vi "LOX Saturation Lookup.vi"(9 "error in":errorcluster, 11 "Temperature":dbl=-280.0) -> (1 "error out":errorcluster, 2 "Saturation Density":dbl, 3 "Saturation Pressure":dbl)   [LabVIEW 2024]
uses:
  <vilib>/Utility/file.llb/Read Delimited Spreadsheet (DBL).vi
panel:
  in  "Lookup Table":dbl[][](array[numeric])=[[-320.0, 3.118, 75.025, 0.013329], [-319.0, 3.3774, 74.862, 0.013358], [-318.0, 3.654, 74.699, 0.013387], [-317.0, 3.9484, 74.536, 0.013416], [-316.0, 4.2615, 74.372, 0.013446], [-315.0, 4.5941, 74.208, 0.013476], [-314.0, 4.9471, 74.044, 0.013506], [-313.0, 5.3214, 73.879, 0.013536], [-312.0, 5.7178, 73.714, 0.013566], [-311.0, 6.1372, 73.548, 0.013597], [-310.0, 6.5807, 73.382, 0.013627], [-309.0, 7.0491, 73.216, 0.013658], [-308.0, 7.5434, 73.049, 0.013689], [-307.0, 8.0646, 72.882, 0.013721], [-306.0, 8.6136, 72.714, 0.013752], [-305.0, 9.1915, 72.546, 0.013784], [-304.0, 9.7994, 72.378, 0.013816], [-303.0, 10.438, 72.209, 0.013849], [-302.0, 11.109, 72.039, 0.013881], [-301.0, 11.813, 71.869, 0.013914], [-300.0, 12.551, 71.699, 0.013947], [-299.0, 13.324, 71.528, 0.013981], [-298.0, 14.134, 71.356, 0.014014], [-297.0, 14.981, 71.184, 0.014048], [-296.0, 15.867, 71.011, 0.014082], [-295.0, 16.793, 70.838, 0.014117], [-294.0, 17.76, 70.664, 0.014151], [-293.0, 18.769, 70.49, 0.014186], [-292.0, 19.821, 70.315, 0.014222], [-291.0, 20.918, 70.139, 0.014257], [-290.0, 22.06, 69.963, 0.014293], [-289.0, 23.25, 69.786, 0.01433], [-288.0, 24.488, 69.608, 0.014366], [-287.0, 25.775, 69.43, 0.014403], [-286.0, 27.113, 69.251, 0.01444], [-285.0, 28.503, 69.072, 0.014478], [-284.0, 29.946, 68.891, 0.014516], [-283.0, 31.444, 68.71, 0.014554], [-282.0, 32.997, 68.529, 0.014592], [-281.0, 34.608, 68.346, 0.014631], [-280.0, 36.276, 68.163, 0.014671], [-279.0, 38.005, 67.978, 0.014711], [-278.0, 39.795, 67.794, 0.014751], [-277.0, 41.647, 67.608, 0.014791], [-276.0, 43.562, 67.421, 0.014832], [-275.0, 45.543, 67.234, 0.014874], [-274.0, 47.59, 67.045, 0.014915], [-273.0, 49.704, 66.856, 0.014958], [-272.0, 51.888, 66.666, 0.015], [-271.0, 54.142, 66.475, 0.015043], [-270.0, 56.468, 66.283, 0.015087], [-269.0, 58.866, 66.09, 0.015131], [-268.0, 61.34, 65.895, 0.015176], [-267.0, 63.889, 65.7, 0.015221], [-266.0, 66.516, 65.504, 0.015266], [-265.0, 69.221, 65.307, 0.015312], [-264.0, 72.006, 65.109, 0.015359], [-263.0, 74.872, 64.909, 0.015406], [-262.0, 77.822, 64.709, 0.015454], [-261.0, 80.855, 64.507, 0.015502], [-260.0, 83.975, 64.304, 0.015551], [-259.0, 87.181, 64.1, 0.015601], [-258.0, 90.476, 63.895, 0.015651], [-257.0, 93.861, 63.688, 0.015701], [-256.0, 97.337, 63.48, 0.015753], [-255.0, 100.91, 63.271, 0.015805], [-254.0, 104.57, 63.06, 0.015858], [-253.0, 108.33, 62.848, 0.015911], [-252.0, 112.18, 62.635, 0.015966], [-251.0, 116.14, 62.42, 0.016021], [-250.0, 120.19, 62.203, 0.016076], [-249.0, 124.35, 61.985, 0.016133], [-248.0, 128.61, 61.766, 0.01619], [-247.0, 132.97, 61.545, 0.016248], [-246.0, 137.44, 61.322, 0.016307], [-245.0, 142.01, 61.097, 0.016367], [-244.0, 146.7, 60.871, 0.016428], [-243.0, 151.49, 60.643, 0.01649], [-242.0, 156.4, 60.413, 0.016553], [-241.0, 161.42, 60.181, 0.016617], [-240.0, 166.56, 59.947, 0.016681], [-239.0, 171.81, 59.711, 0.016747], [-238.0, 177.18, 59.473, 0.016814], [-237.0, 182.67, 59.233, 0.016883], [-236.0, 188.28, 58.991, 0.016952], [-235.0, 194.01, 58.746, 0.017022], [-234.0, 199.86, 58.499, 0.017094], [-233.0, 205.85, 58.25, 0.017167], [-232.0, 211.96, 57.998, 0.017242], [-231.0, 218.19, 57.743, 0.017318], [-230.0, 224.56, 57.486, 0.017395], [-229.0, 231.06, 57.226, 0.017474], [-228.0, 237.7, 56.964, 0.017555], [-227.0, 244.47, 56.698, 0.017637], [-226.0, 251.37, 56.429, 0.017721], [-225.0, 258.42, 56.157, 0.017807], [-224.0, 265.6, 55.882, 0.017895], [-223.0, 272.93, 55.603, 0.017985], [-222.0, 280.4, 55.321, 0.018076], [-221.0, 288.02, 55.035, 0.01817], [-220.0, 295.78, 54.745, 0.018266], [-219.0, 303.69, 54.451, 0.018365], [-218.0, 311.75, 54.153, 0.018466], [-217.0, 319.97, 53.85, 0.01857], [-216.0, 328.34, 53.543, 0.018677], [-215.0, 336.87, 53.231, 0.018786], [-214.0, 345.55, 52.914, 0.018899], [-213.0, 354.4, 52.591, 0.019015], [-212.0, 363.41, 52.263, 0.019134], [-211.0, 372.58, 51.929, 0.019257], [-210.0, 381.92, 51.588, 0.019384], [-209.0, 391.42, 51.241, 0.019515], [-208.0, 401.1, 50.887, 0.019651], [-207.0, 410.95, 50.526, 0.019792], [-206.0, 420.98, 50.156, 0.019938], [-205.0, 431.18, 49.778, 0.020089], [-204.0, 441.57, 49.39, 0.020247], [-203.0, 452.13, 48.993, 0.020411], [-202.0, 462.88, 48.586, 0.020582], [-201.0, 473.82, 48.167, 0.020761], [-200.0, 484.95, 47.736, 0.020949]]
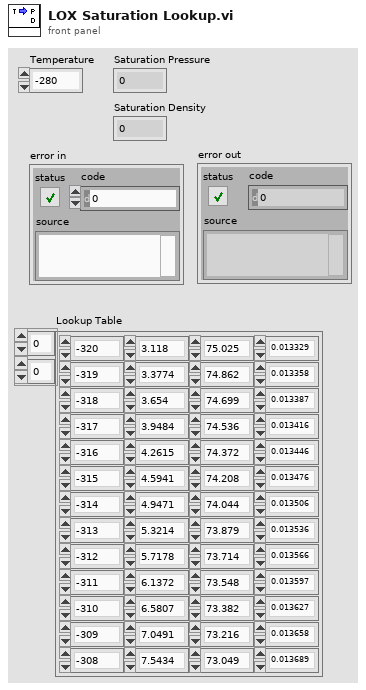
[diagram p1: front panel]
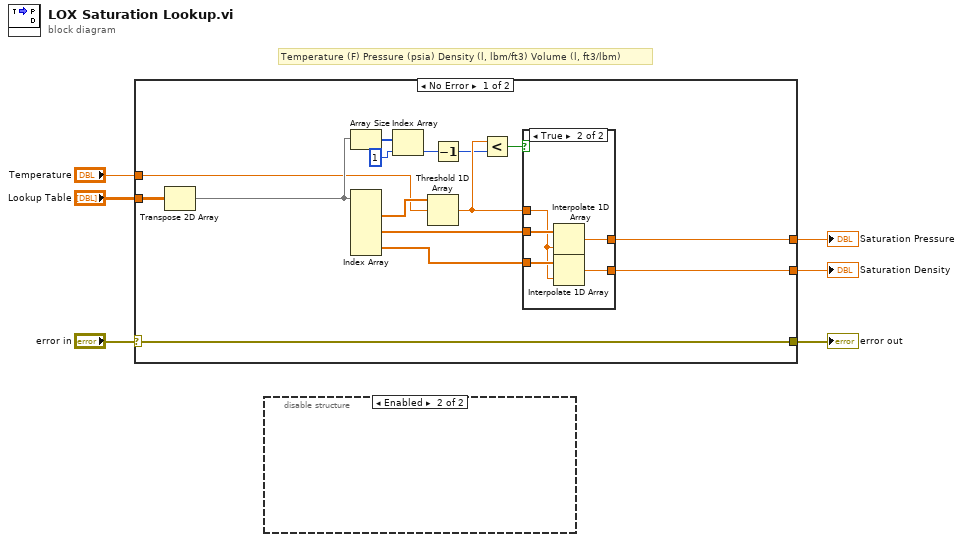
[diagram p0: block diagram]
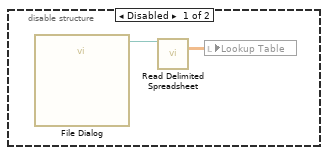
[diagram p2: hidden frame]
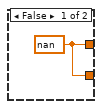
[diagram p3: hidden frame]
diagram:
  # "Temperature (F)\tPressure (psia)\tDensity (l, lbm/ft3)\tVolume (l, ft3/lbm)"
  n1 = case shown="No Error" "error in" {
    selector: "error in" -> [w21 w28]
    tunnel: [w21 w28] -> w5
    tunnel: "Temperature" -> [w9 _]
    tunnel: [w8 _] -> w3
    tunnel: "Lookup Table" -> [w20 _]
    tunnel: [w7 _] -> w1
    frame No Error {
      n2 = Transpose 2D Array(2D array=w20) -> (transposed array=w10:dbl[][])
      n3 = Array Size(array=w10) -> (size(s)=w17:i32[])
      n4 = Index Array(array=w10) -> (element #1=w19:dbl[], element #2=w18:dbl[], element #3=w11:dbl[])  [unwired: 6 in]
      n5 = Index Array(array=w17, index=1) -> (element=w16:i32)
      n6 = Threshold 1D Array(2:w9, 3:w19) -> (0:w15:dbl)  [unwired: 1 in]
      n7 = Decrement(x=w16) -> (x-1=w12:i32)
      n8 = Less?(x=w15, y=w12) -> (x < y?=w14:bool)
      n9 = case shown="True" w14 {
        tunnel: w18 -> [_ w27]
        tunnel: [w22 w26] -> w8
        tunnel: w15 -> [_ w24]
        tunnel: w11 -> [_ w25]
        tunnel: [w22 w23] -> w7
        frame False {
          w22 = nan
        }
        frame True {
          n10 = Interpolate 1D Array(1:w24, 2:w27) -> (0:w26:dbl)
          n11 = Interpolate 1D Array(1:w24, 2:w25) -> (0:w23:dbl)
        }
      }
    }
    frame Error {
    }
  }
  "Saturation Pressure" <- w3
  "error out" <- w5
  "Saturation Density" <- w1
  n12 = disable-structure shown="Enabled" {
    frame Disabled {
      n13 = call "File Dialog"() -> ("selected path"=w29:path)  [unwired: 12 in, 3 out]
      n14 = call-poly <vilib>:"Read Delimited Spreadsheet.vi"("file path (dialog if empty)"=w29) -> ("all rows"=w30:dbl[][])  [unwired: 9 in, 5 out]
      n15 = local write "Lookup Table"(w30) -> ()
    }
    frame Enabled {
    }
  }
